vi "构造类实例（数据采集接口）.vi"(8 "error in (no error)":errorcluster caption="错误输入（无错误）") -> (0 "error out":errorcluster caption="错误输出")   [LabVIEW 2011]
panel:
  out "数据采集 输出":refnum<class "数据采集.lvclass"> caption="DNL_LabVIEW Object out"
  in  "数据采集 输入":refnum<class "数据采集.lvclass"> caption="DNL_LabVIEW Object in"
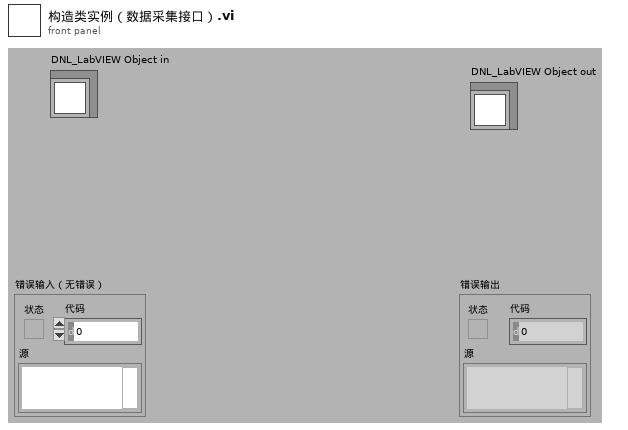
[diagram p1: front panel]
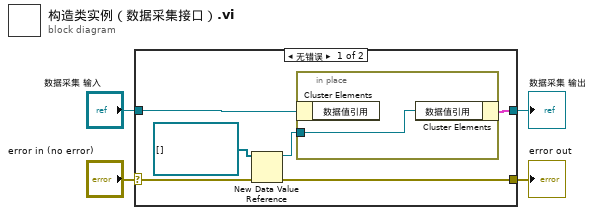
[diagram p0: block diagram]
diagram:
  n1 = case shown="无错误" "error in (no error)" {
    selector: "error in (no error)" -> [w6 w13]
    tunnel: [w5 w13] -> w3
    tunnel: [w7 w12] -> w1
    tunnel: "数据采集 输入" -> [w9 w12]
    frame No Error {
      n2 = New Data Value Reference(data value=refnum<class "订阅者接口.lvclass">[] [], error in=w6) -> (data value reference=w8:refnum<data-value>, error out=w5:errorcluster)
      n3 = in-place {
        in-place-border: w8 -> [w11]
        n4 = in-place-cluster #1(w9) -> ()  [unwired: 1 out]
        n5 = in-place-cluster #1("数据值引用"=w11) -> (w7:cluster{})
      }
    }
    frame Error {
    }
  }
  "error out" <- w3
  "数据采集 输出" <- w1
